vi "VI Stopped Logic - For test.vi"(8 "Error In":errorcluster, 9 "THIS VI State IN":T1, 10 "Signalling VI State IN":T1, 11 "Heartbeat Event Types IN":T2=enum."Timeout") -> (0 "Error Out":errorcluster, 1 "THIS VI State OUT":T1, 3 "Set HFG?":bool)   [LabVIEW 2012]
doc: "SciScan 1.2 160622\nThis VI implements the logic to set the HFG variable if the MASTER or SLAVE VI transitions between 'VI Stopped' and 'VI running'"
uses:
  Custom Controls/Heartbeat_States.ctl
  Custom Controls and Typedefs/Heartbeat Event Source.ctl
panel:
  in  "Signalling VI Name":string
  in  "Masters and Slaves":cluster{"Slaves":string[], "Masters":string[]}
  out "Slave Stopped":bool
  out "Master Stopped":bool
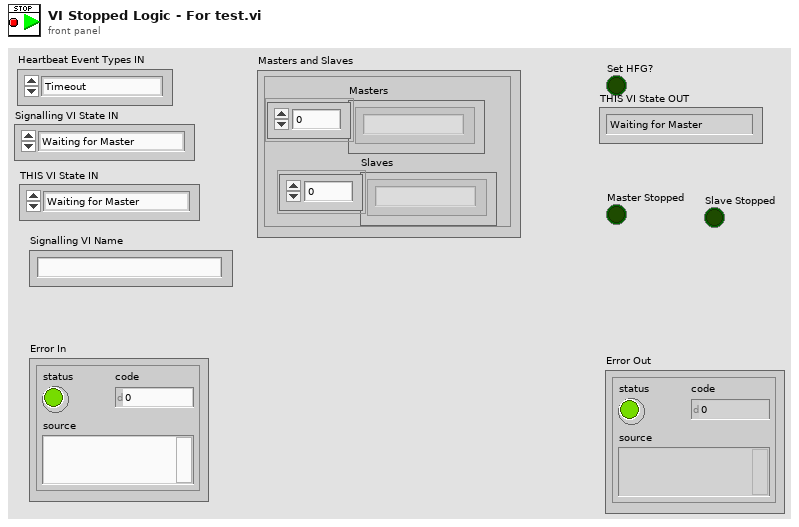
[diagram p1: front panel]
types:
  T1 = typedef "Heartbeat_States.ctl" = enum16{"Waiting for Master", "Instruction Issued", "Waiting for Slave Completion", "Completed", "Cancelled", "Failed", "Broken Link"}
  T2 = typedef "Heartbeat Event Source.ctl" = enum16{"Unknown Source", "Timeout", "This VI", "Master", "Slave"}
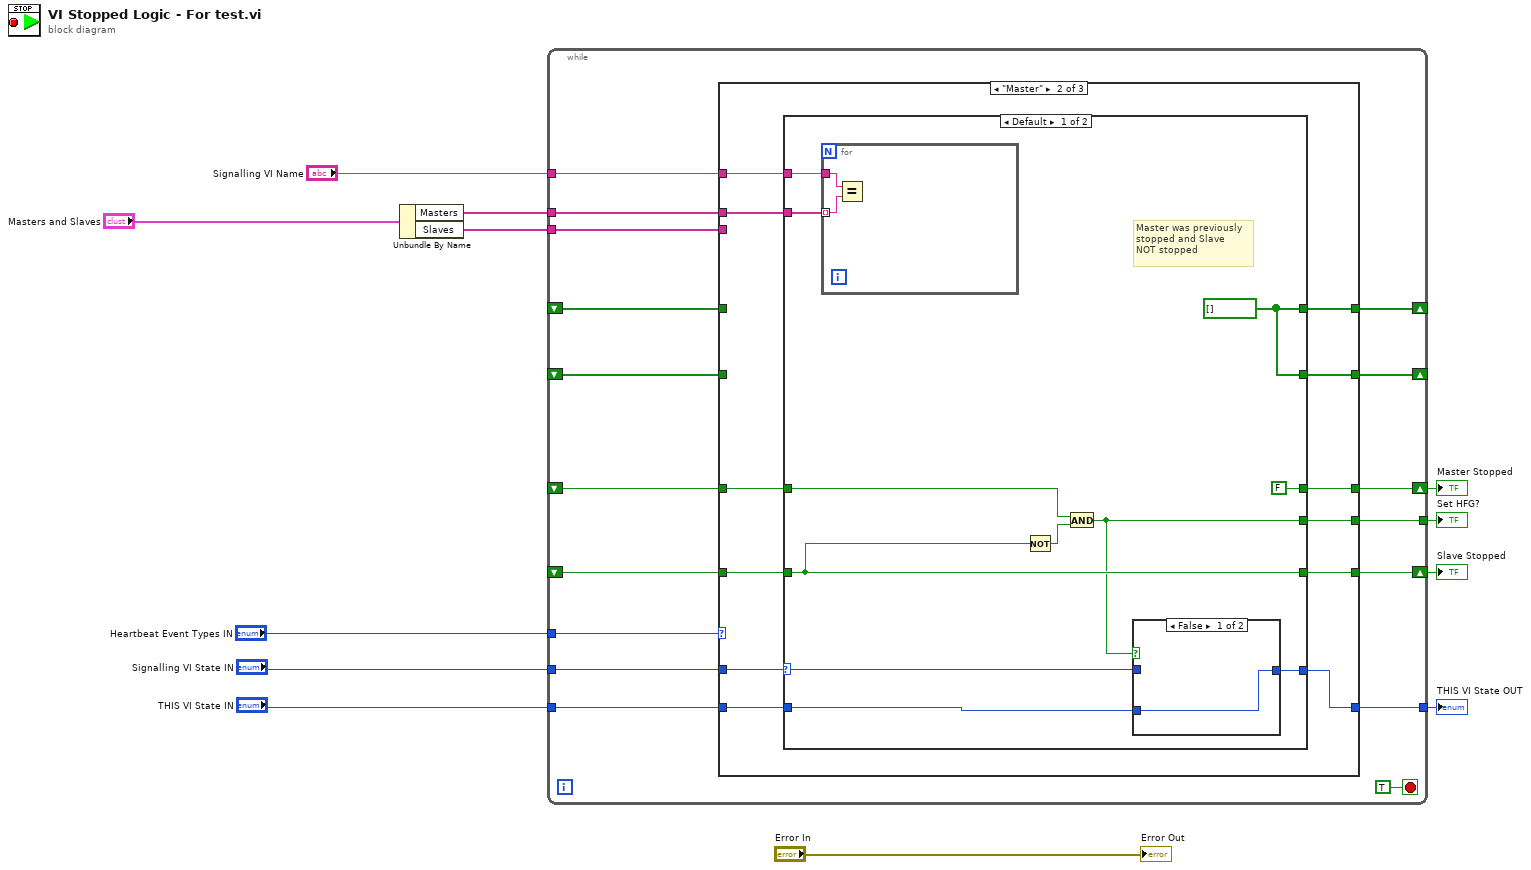
[diagram p0: block diagram]
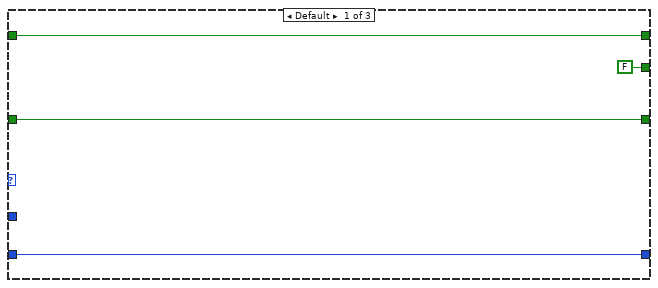
[diagram p2: hidden frame]
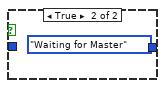
[diagram p3: hidden frame]
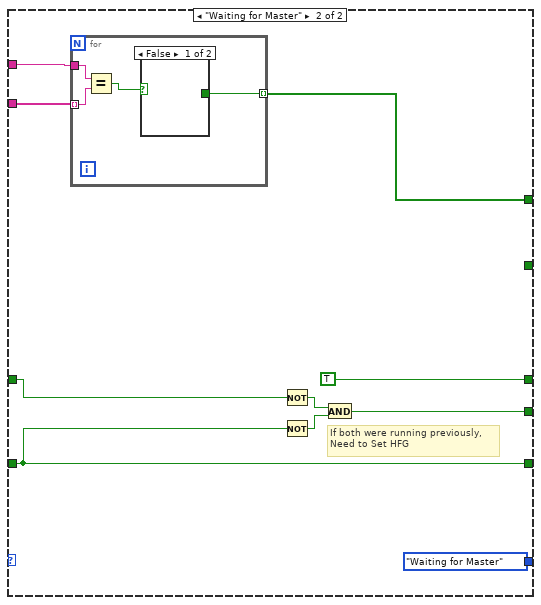
[diagram p4: hidden frame]
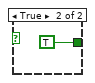
[diagram p5: hidden frame]
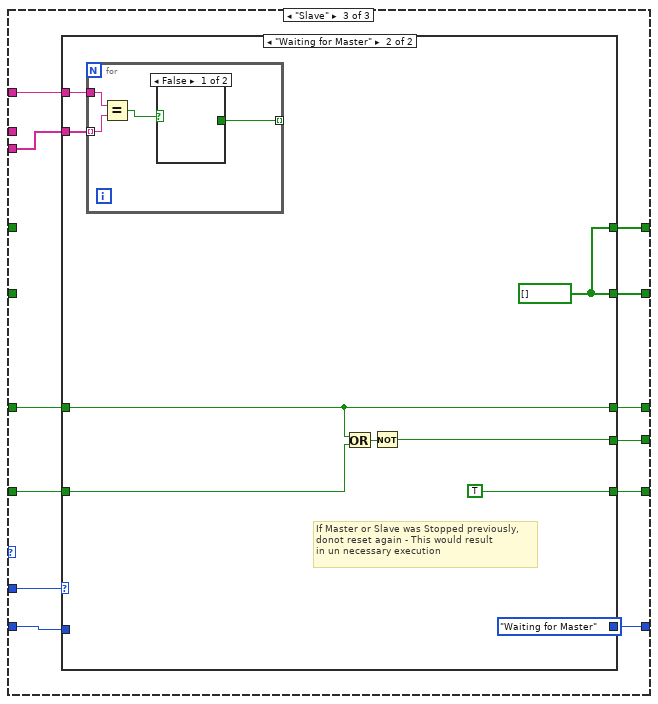
[diagram p6: hidden frame]
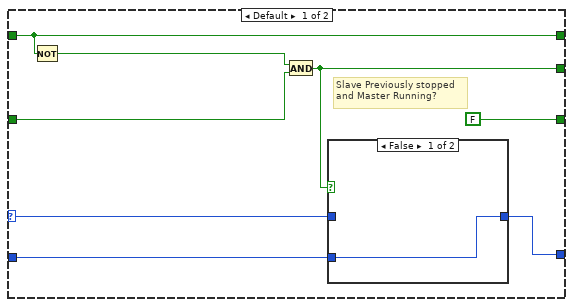
[diagram p7: hidden frame]
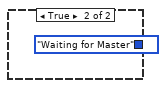
[diagram p8: hidden frame]
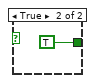
[diagram p9: hidden frame]
diagram:
  n1 = Unbundle By Name("Masters and Slaves") -> ("Masters"=w3:string[], "Slaves"=w2:string[])
  n2 = while {
    shift-right: [w28] -> w8
    shift-left: _ -> [w26]
    shift-right: [w27] -> w9
    shift-left: _ -> [w25]
    tunnel: [w24] -> w12
    tunnel: [w23] -> w11
    tunnel: "THIS VI State IN" -> [w22]
    tunnel: "Signalling VI State IN" -> [w21]
    tunnel: "Heartbeat Event Types IN" -> [w20]
    tunnel: w3 -> [w19]
    tunnel: w2 -> [w18]
    tunnel: "Signalling VI Name" -> [w17]
    shift-right: [w16] -> _
    shift-left: _ -> [w15]
    shift-right: [w14] -> _
    shift-left: _ -> [w13]
    stop <- TRUE stop-if-true
    n3 = case shown="\"Master\"" w20 {
      tunnel: w21 -> [_ w45 w87]
      tunnel: [w32 w41 w86] -> w28
      tunnel: [w31 w44 w84] -> w27
      tunnel: w26 -> [w32 w43 w83]
      tunnel: w25 -> [w31 w42 w85]
      tunnel: [FALSE w40 w82] -> w24
      tunnel: [w30 w39 w81] -> w23
      tunnel: w22 -> [w30 w38 w80]
      tunnel: w19 -> [_ w37 _]
      tunnel: w18 -> [_ _ w78]
      tunnel: w17 -> [_ w36 w79]
      tunnel: [_ w35 w76] -> w16
      tunnel: w15 -> [_ _ _]
      tunnel: [_ w34 w77] -> w14
      tunnel: w13 -> [_ _ _]
      frame Default {
      }
      frame "Master" {
        n4 = case shown="Default" w45 {
          selector: w45 -> [w50 _]
          tunnel: [FALSE TRUE] -> w44
          tunnel: w43 -> [w54 w67]
          tunnel: w42 -> [w56 w68]
          tunnel: [w54 w67] -> w41
          tunnel: [w52 w64] -> w40
          tunnel: [w51 Heartbeat_States."Waiting for Master" ("VI State")] -> w39
          tunnel: w38 -> [w49 _]
          tunnel: w37 -> [w48 w62]
          tunnel: w36 -> [w47 w63]
          tunnel: [w46 w61] -> w35
          tunnel: [w46 _] -> w34
          frame Default {
            w46 = bool[] []
            # "Master was previously\nstopped and Slave\nNOT stopped"
            n5 = for {
              tunnel: w48 -> [w57] mode=indexing
              tunnel: w47 -> [w58]
              n6 = Equal?(x=w58, y=w57) -> ()  [unwired: 1 out]
            }
            n7 = Not(x=w54) -> (.not. x?=w53:bool)
            n8 = And(x=w56, y=w53) -> (x .and. y?=w52:bool)
            n9 = case shown="False" w52 {
              tunnel: [w59 Heartbeat_States."Waiting for Master" ("VI State")] -> w51
              tunnel: w50 -> [_ _]
              tunnel: w49 -> [w59 _]
              frame False {
              }
              frame True {
              }
            }
          }
          frame "Waiting for Master" {
            # "If both were running previously,\nNeed to Set HFG"
            n10 = for {
              tunnel: w62 -> [w73] mode=indexing
              tunnel: w63 -> [w74]
              tunnel: [w71] -> w61 mode=indexing
              n11 = Equal?(x=w74, y=w73) -> (x = y?=w72:bool)
              n12 = case shown="False" w72 {
                tunnel: [_ TRUE] -> w71
                frame False {
                }
                frame True {
                }
              }
            }
            n13 = Not(x=w68) -> (.not. x?=w66:bool)
            n14 = Not(x=w67) -> (.not. x?=w65:bool)
            n15 = And(x=w66, y=w65) -> (x .and. y?=w64:bool)
          }
        }
      }
      frame "Slave" {
        n16 = case shown="\"VI stopped\"" w87 {
          selector: w87 -> [w90 _]
          tunnel: [FALSE TRUE] -> w86
          tunnel: w85 -> [w92 w105]
          tunnel: [w92 w105] -> w84
          tunnel: w83 -> [w94 w104]
          tunnel: [w91 w102] -> w82
          tunnel: [w89 Heartbeat_States."Waiting for Master" ("VI State")] -> w81
          tunnel: w80 -> [w88 _]
          tunnel: w79 -> [_ w100]
          tunnel: w78 -> [_ w99]
          tunnel: [_ w98] -> w77
          tunnel: [_ w98] -> w76
          frame Default {
            # "Slave Previously stopped\nand Master Running?"
            n17 = Not(x=w92) -> (.not. x?=w93:bool)
            n18 = And(x=w93, y=w94) -> (x .and. y?=w91:bool)
            n19 = case shown="False" w91 {
              tunnel: w90 -> [_ _]
              tunnel: [w96 Heartbeat_States."Waiting for Master" ("VI State")] -> w89
              tunnel: w88 -> [w96 _]
              frame False {
              }
              frame True {
              }
            }
          }
          frame "Waiting for Master" {
            w98 = bool[] []
            # "If Master or Slave was Stopped previously,\ndonot reset again - This would result\nin un necessary execution"
            n20 = for {
              tunnel: w99 -> [w109] mode=indexing
              tunnel: w100 -> [w110]
              tunnel: [w107] -> _ mode=indexing
              n21 = Equal?(x=w110, y=w109) -> (x = y?=w108:bool)
              n22 = case shown="False" w108 {
                tunnel: [_ TRUE] -> w107
                frame False {
                }
                frame True {
                }
              }
            }
            n23 = Or(x=w105, y=w104) -> (x .or. y?=w103:bool)
            n24 = Not(x=w103) -> (.not. x?=w102:bool)
          }
        }
      }
    }
  }
  "Set HFG?" <- w12
  "THIS VI State OUT" <- w11
  "Master Stopped" <- w9
  "Slave Stopped" <- w8
  "Error Out" <- "Error In"
